vi "Actor Core.vi"(8 "error in":errorcluster, 11 "For Loop Dialog In":refnum<class "Test Step Dialog.lvclass">) -> (0 "error out":errorcluster, 3 "Actor out":refnum<class "Actor.lvclass">)   [LabVIEW 2017, in "Test Step Dialog.lvclass"]
doc: "(<B>Filename</B>: Actor Framework.lvlib:Actor.lvclass:Actor Core.vi)\n\nReceives messages to the actor, reacts to them, and initiates any error handling that may shut the actor down.\n\nDescendant classes may override this VI to append parallel tasks for the actor to complete while it handles messages. Overrides use the Call Parent Method node.\n\n<License>\nCopyright © 2017 Composed Systems, LLC | All rights reserved\nwww.composed.io\n\nAuthor: Ethan Stern <ethan.stern@composed.io>\n\nThis software is provided \"AS IS\" WITHOUT WARRANTIES, either express or implied, AND IS FOR EDUCATIONAL PURPOSES ONLY.\n</License>"
uses:
  Test Step Dialog.lvclass
  ITest Executive Builder Dialog/ITest Executive Builder Dialog.lvclass
  <vilib>/gpm_packages/@cs/mva-viewable/Source/ActorEvents/IEventAggregator/IEventAggregator.lvclass
  <vilib>/event_ctls.llb/lveventtype.ctl
  C:/Users/jonmc/Documents/Git/Test Executive Builder/Source/Test Executive Builder Dialogs/ITest Executive Builder Dialog/ITest Executive Builder Dialog.lvclass
  C:/Users/jonmc/Documents/Git/Test Executive Builder/gpm_packages/@cs/mva-viewable/Source/ActorEvents/IEventAggregator/IEventAggregator.lvclass
  <vilib>/gpm_packages/@cs/mva-viewable/Source/IViewable/ProtectedSubpanel/ProtectedSubpanel.lvclass
  <vilib>/ActorFramework/Actor/Actor.lvclass
panel:
  in  "Tab Control":enum32{"Value", "Pointer"}(tab)
  in  "Flatten Pointer":bool caption="Flatten?"
  in  "Pointer":u16(ring)
  in  "Attribute Notes":string
  in  "Attribute Name":u16(ring)
  in  "Cancel":bool
  in  "OK":bool
  in  "Name":string
  # "Edit Test Step"
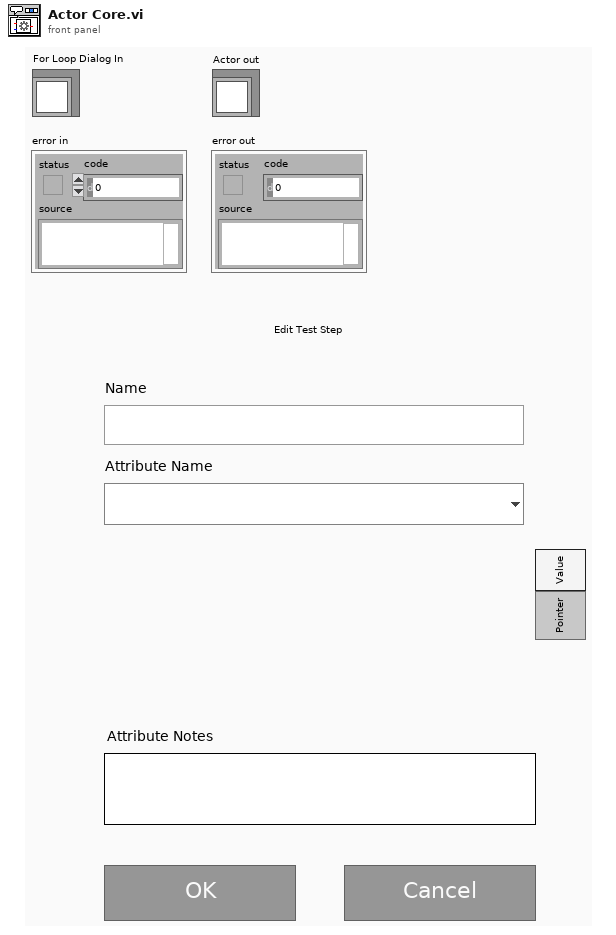
[diagram p1: front panel]
types:
  T1 = typedef "lveventtype.ctl" = enum32{"Null", "Timeout", "Annotation Menu Selection", "Annotation Menu Selection?", "App Instance Close", "App Instance Close?", "Autoscale Range Change", "Bookmark Info Change", "Cell Edit", "Cell Edit?", "Cursor Grab", "Cursor Grab?", "Cursor Menu Selection", "Cursor Menu Selection?", "Cursor Move", "Cursor Release", "Data Change", "Direction Change", "Display State Change", "Drag Ended", "Drag Enter", "Drag Leave", "Drag Over", "Drag Source Update", "Drag Starting", "Drag Starting?", "Drop", "Exec State Change", "Key Down", "Key Down?", "Key Repeat", "Key Repeat?", "Key Up", "Listbox Double Click", "Menu Activation?", "Menu Selection (App)", "Menu Selection? (App)", "Menu Selection (User)", "Mouse Down", "Mouse Down?", "Mouse Enter", "Mouse Leave", "Mouse Move", "Mouse Up", "Mouse Wheel", "NI Security User Change (App)", "Pane Size", "Panel Close", "Panel Close?", "Panel Resize", "Plot Attribute Change", "Scale Range Change", "Shortcut Menu Activation?", "Shortcut Menu Selection (App)", "Shortcut Menu Selection? (App)", "Shortcut Menu Selection (User)", "Tree Double Click", "Tree Drag", "Tree Drag?", "Tree Drop", "Tree Drop?", "Tree Item Close", "Tree Item Close?", "Tree Item Open", "Tree Item Open?", "User Event", "Value Change"}
  T2 = typedef "IViewable.lvlib/ProtectedSubpanel.lvclass/Protected Subpanel Reference.ctl" = refnum<data-value>
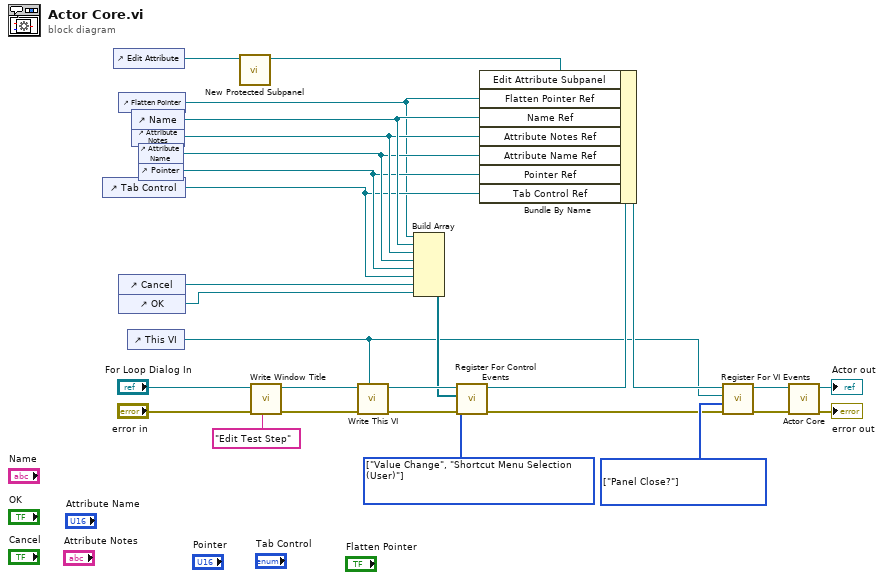
[diagram p0: block diagram]
diagram:
  w16 = T1[] [enum."Panel Close?"] items=["Null", "Timeout", "Annotation Menu Selection", "Annotation Menu Selection?", "App Instance Close", "App Instance Close?", "Autoscale Range Change", "Bookmark Info Change", "Cell Edit", "Cell Edit?", "Cursor Grab", "Cursor Grab?", "Cursor Menu Selection", "Cursor Menu Selection?", "Cursor Move", "Cursor Release", "Data Change", "Direction Change", "Display State Change", "Drag Ended", "Drag Enter", "Drag Leave", "Drag Over", "Drag Source Update", "Drag Starting", "Drag Starting?", "Drop", "Exec State Change", "Key Down", "Key Down?", "Key Repeat", "Key Repeat?", "Key Up", "Listbox Double Click", "Menu Activation?", "Menu Selection (App)", "Menu Selection? (App)", "Menu Selection (User)", "Mouse Down", "Mouse Down?", "Mouse Enter", "Mouse Leave", "Mouse Move", "Mouse Up", "Mouse Wheel", "NI Security User Change (App)", "Pane Size", "Panel Close", "Panel Close?", "Panel Resize", "Plot Attribute Change", "Scale Range Change", "Shortcut Menu Activation?", "Shortcut Menu Selection (App)", "Shortcut Menu Selection? (App)", "Shortcut Menu Selection (User)", "Tree Double Click", "Tree Drag", "Tree Drag?", "Tree Drop", "Tree Drop?", "Tree Item Close", "Tree Item Close?", "Tree Item Open", "Tree Item Open?", "User Event", "Value Change"] ("Registration Types")
  w21 = T1[] [enum."Value Change", enum."Shortcut Menu Selection (User)"] items=["Null", "Timeout", "Annotation Menu Selection", "Annotation Menu Selection?", "App Instance Close", "App Instance Close?", "Autoscale Range Change", "Bookmark Info Change", "Cell Edit", "Cell Edit?", "Cursor Grab", "Cursor Grab?", "Cursor Menu Selection", "Cursor Menu Selection?", "Cursor Move", "Cursor Release", "Data Change", "Direction Change", "Display State Change", "Drag Ended", "Drag Enter", "Drag Leave", "Drag Over", "Drag Source Update", "Drag Starting", "Drag Starting?", "Drop", "Exec State Change", "Key Down", "Key Down?", "Key Repeat", "Key Repeat?", "Key Up", "Listbox Double Click", "Menu Activation?", "Menu Selection (App)", "Menu Selection? (App)", "Menu Selection (User)", "Mouse Down", "Mouse Down?", "Mouse Enter", "Mouse Leave", "Mouse Move", "Mouse Up", "Mouse Wheel", "NI Security User Change (App)", "Pane Size", "Panel Close", "Panel Close?", "Panel Resize", "Plot Attribute Change", "Scale Range Change", "Shortcut Menu Activation?", "Shortcut Menu Selection (App)", "Shortcut Menu Selection? (App)", "Shortcut Menu Selection (User)", "Tree Double Click", "Tree Drag", "Tree Drag?", "Tree Drop", "Tree Drop?", "Tree Item Close", "Tree Item Close?", "Tree Item Open", "Tree Item Open?", "User Event", "Value Change"] ("Registration Types")
  n1 = control-ref of="Tab Control"() -> (w4:refnum<vi>)
  n2 = control-ref of="Edit Attribute"() -> (w3:refnum<vi>)
  n3 = control-ref of="Flatten Pointer"() -> (w1:refnum<vi>)
  n4 = control-ref of="Cancel"() -> (w20:refnum<vi>)
  n5 = control-ref of="OK"() -> (w19:refnum<vi>)
  n6 = control-ref of="This VI"() -> (w11:refnum<vi>)
  n7 = control-ref of="Name"() -> (w18:refnum<vi>)
  n8 = control-ref of="Attribute Notes"() -> (w7:refnum<vi>)
  n9 = control-ref of="Attribute Name"() -> (w6:refnum<vi>)
  n10 = control-ref of="Pointer"() -> (w5:refnum<vi>)
  n11 = call <vilib>:"New Protected Subpanel.vi"("SubPnl Refnum"=w3) -> ("Protected Subpanel"=w2:T2)  [unwired: 9 in, 1 out]
  n12 = call "Write Window Title.vi"("Window Title"="Edit Test Step", "ITest Executive Builder Dialog in"="For Loop Dialog In") -> ("ITest Executive Builder Dialog out"=w9:refnum<class "Test Step Dialog.lvclass">)  [unwired: 9 in]
  n13 = call "Write This VI.vi"("This VI"=w11, "ITest Executive Builder Dialog in"=w9) -> ("ITest Executive Builder Dialog out"=w23:refnum<class "Test Step Dialog.lvclass">)  [unwired: 9 in]
  n14 = Build Array(w1, w18, w7, w6, w5, w4, w20, w19) -> (w17:refnum<vi>[])
  n15 = call <vilib>:"Register For Control Events.vi"("error in (no error)"="error in", "Registration Types"=w21, "Control Refnums"=w17, "IEventAggregator In"=w23) -> ("error out"=w15:errorcluster, "IEventAggregator Out"=w22:refnum<class "Test Step Dialog.lvclass">)  [unwired: 6 in]
  n16 = Bundle By Name(cluster=w22, "Edit Attribute Subpanel"=w2, "Flatten Pointer Ref"=w1, "Name Ref"=w18, "Attribute Notes Ref"=w7, "Attribute Name Ref"=w6, "Pointer Ref"=w5, "Tab Control Ref"=w4) -> (w13:refnum<class "Test Step Dialog.lvclass">)
  n17 = call <vilib>:"Register For VI Events.vi"("error in (no error)"=w15, "Registration Types"=w16, "VI Refnum"=w11, "IEventAggregator In"=w13) -> ("error out"=w14:errorcluster, "IEventAggregator Out"=w12:refnum<class "Test Step Dialog.lvclass">)  [unwired: 6 in]
  n18 = call-parent "Actor Core.vi"("error in"=w14, "ITest Executive Builder Dialog In"=w12) -> ("error out"=→"error out":errorcluster, "Actor out"=→"Actor out":refnum<class "Actor.lvclass">)  [unwired: 8 in]
